vi "BuildBooleanWave.vi"(0 "DAQmx Global Channel":refnum<k21>, 1 "Ctrl_Signal":T1, 2 "TS RefShot":bool, 3 "error in (no error)":errorcluster) -> (6 "waveform out":digitalwaveform(waveform)={"t0"=timestamp(0 s since 1904-01-01), "dt"=1.0, "Y"={"transitions"=[], "data"=[]}}, 9 "error out":errorcluster)   [LabVIEW 2016]
uses:
  Ctrl_Signal.ctl
  <vilib>/Waveform/DWDTOps.llb/DWDT Boolean Array to Digital.vi
  <resource>/objmgr/daqmx.rc
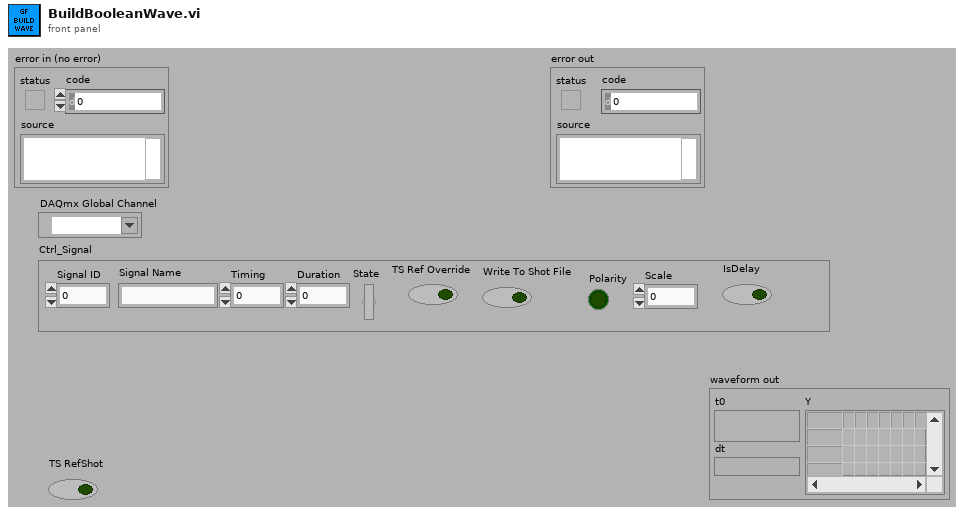
[diagram p1: front panel]
types:
  T1 = typedef "Ctrl_Signal.ctl" = cluster{"Signal Name":string, "Timing":dbl, "Duration":dbl, "State":bool, "TS Ref Override":bool, "Write To Shot File":bool, "Polarity":bool, "Signal ID":dbl, "Scale":dbl, "IsDelay":bool}
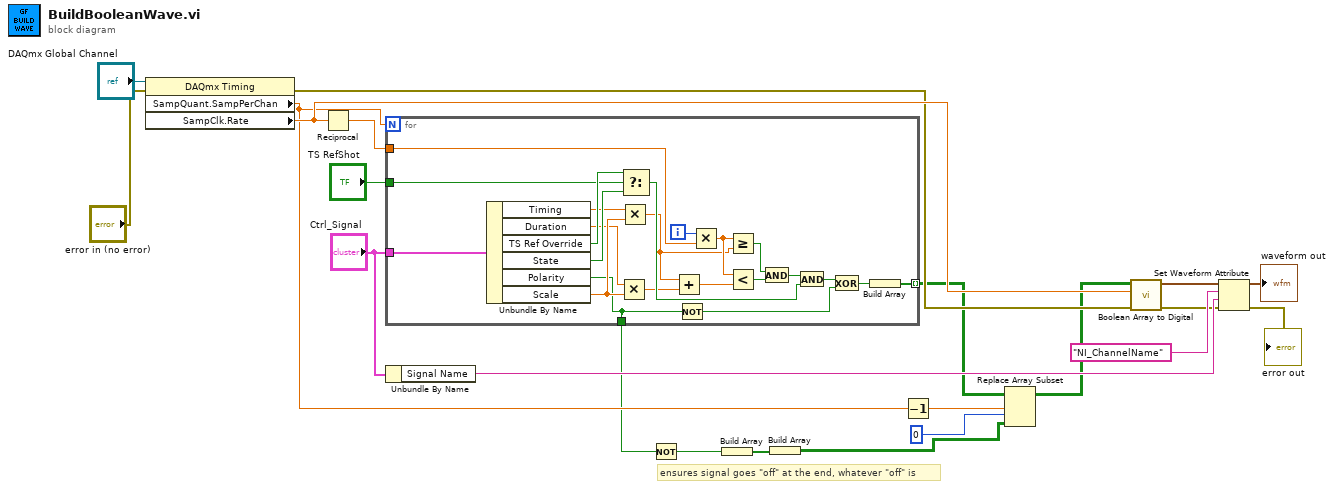
[diagram p0: block diagram]
diagram:
  # "ensures signal goes \"off\" at the end, whatever \"off\" is"
  n1 = property class="DAQmx Timing"(reference="DAQmx Global Channel", error in="error in (no error)") -> (error out=w11:errorcluster, "SampQuant.SampPerChan"=w5:dbl, "SampClk.Rate"=w14:dbl)  [unwired: 1 out]
  n2 = Reciprocal(x=w14) -> (1/x=w17:dbl)
  n3 = for {
    N: w5 -> [_]
    tunnel: w17 -> [w43]
    tunnel: "Ctrl_Signal" -> [w42]
    tunnel: "TS RefShot" -> [w36]
    tunnel: [w31] -> w9 mode=indexing
    tunnel: [w23] -> w1
    i -> [w44]
    n4 = Unbundle By Name(w42) -> ("Timing"=w27:dbl, "Duration"=w28:dbl, "TS Ref Override"=w38:bool, "State"=w37:bool, "Polarity"=w23:bool, "Scale"=w29:dbl)
    n5 = Multiply(x=w28, y=w29) -> (x*y=w25:dbl)
    n6 = Multiply(x=w27, y=w29) -> (x*y=w26:dbl)
    n7 = Select(t=w38, s=w36, f=w37) -> (s? t:f=w34:bool)
    n8 = Add(x=w26, y=w25) -> (x+y=w41:dbl)
    n9 = Not(x=w23) -> (.not. x?=w24:bool)
    n10 = Multiply(x=w44, y=w43) -> (x*y=w30:dbl)
    n11 = Greater Or Equal?(x=w30, y=w26) -> (x >= y?=w40:bool)
    n12 = Less?(x=w30, y=w41) -> (x < y?=w39:bool)
    n13 = And(x=w40, y=w39) -> (x .and. y?=w35:bool)
    n14 = And(x=w35, y=w34) -> (x .and. y?=w33:bool)
    n15 = Exclusive Or(1:w24, 2:w33) -> (0:w32:bool)
    n16 = Build Array(w32) -> (w31:bool[])
  }
  n17 = Unbundle By Name("Ctrl_Signal") -> ("Signal Name"=w18:string)
  n18 = Not(x=w1) -> (.not. x?=w2:bool)
  n19 = Build Array(w2) -> (w4:bool[])
  n20 = Build Array(w4) -> (w3:bool[][])
  n21 = Decrement(x=w5) -> (x-1=w6:dbl)
  n22 = Replace Array Subset(array=w9, new element=w3, index (row)=w6, index (col)=0 ("disabled index (col)")) -> (w8:bool[][])
  n23 = call-poly <vilib>:"Boolean Array to Digital.vi"("error in (no error)"=w11, "sample rate"=w14, "boolean array"=w8) -> ("error out"=w13:errorcluster, "digital waveform"=w15:digitalwaveform)  [unwired: 7 in]
  n24 = Set Waveform Attribute(4:w13, 5:w18, 6:"NI_ChannelName" ("name"), 7:w15) -> (0:→"error out":errorcluster, 3:→"waveform out":digitalwaveform)  [unwired: 1 out]
